vi "Auto Aim.vi"() -> ()   [LabVIEW 2020]
panel:
  out "Bottom Motor":dbl
  out "Top Motor":dbl
  out "Reference":dbl[](array[numeric])
  out "Percent":dbl
  out "Index":i32
  out "Closest":dbl
  in  "Distance":dbl
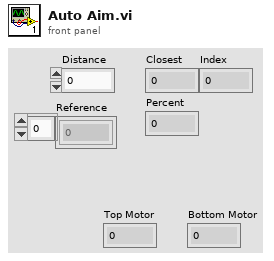
[diagram p1: front panel]
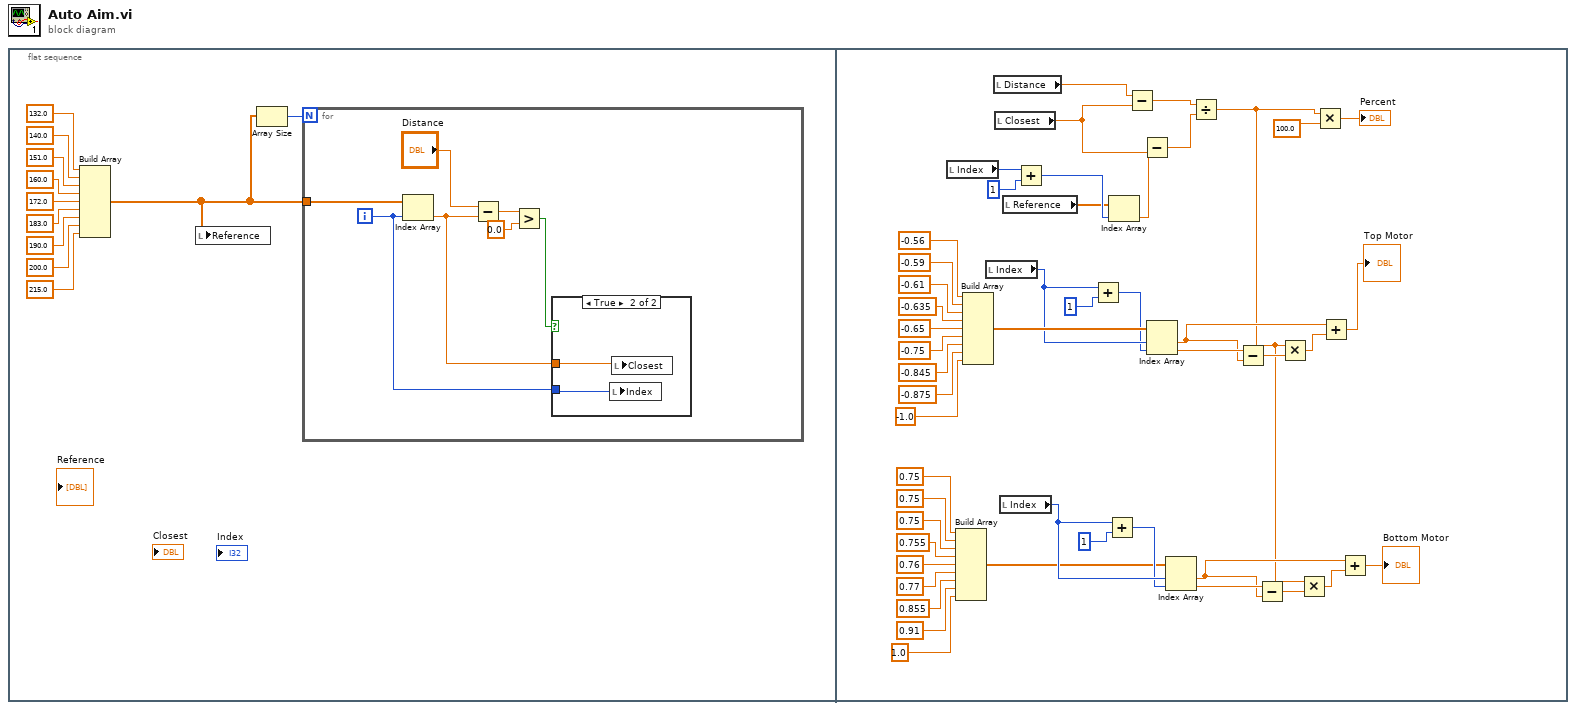
[diagram p0: block diagram]
diagram:
  n1 = flat-sequence {
    frame #0 {
      n2 = Build Array(132.0 ("element"), 140.0 ("element"), 151.0 ("element"), 160.0 ("element"), 172.0 ("element"), 183.0 ("element"), 190.0 ("element"), 200.0 ("element"), 215.0 ("element")) -> (w1:dbl[])
      n3 = local write "Reference"(w1) -> ()
      n4 = Array Size(array=w1) -> (size(s)=w2:i32)
      n5 = for {
        N: w2 -> [_]
        tunnel: w1 -> [w18]
        i -> [w12]
        n6 = Index Array(array=w18, index=w12) -> (element=w13:dbl)
        n7 = Subtract(x="Distance", y=w13) -> (x-y=w17:dbl)
        n8 = Greater?(x=w17, y=0.0) -> (0:w14:bool)
        n9 = case shown="True" w14 {
          tunnel: w13 -> [_ w20]
          tunnel: w12 -> [_ w19]
          frame False {
          }
          frame True {
            n10 = local write "Index"(w19) -> ()
            n11 = local write "Closest"(w20) -> ()
          }
        }
      }
    }
    frame #1 {
      n12 = local read "Index"() -> (w58:i32)
      n13 = Build Array(0.75 ("element"), 0.75 ("element"), 0.75 ("element"), 0.755 ("element"), 0.76 ("element"), 0.77 ("element"), 0.855 ("element"), 0.91 ("element"), 1.0 ("element")) -> (w25:dbl[])
      n14 = Build Array(-0.56 ("element"), -0.59 ("element"), -0.61 ("element"), -0.635 ("element"), -0.65 ("element"), -0.75 ("element"), -0.845 ("element"), -0.875 ("element"), -1.0 ("element")) -> (w50:dbl[])
      n15 = local read "Index"() -> (w48:i32)
      n16 = local read "Distance"() -> (w59:dbl)
      n17 = local read "Closest"() -> (w52:dbl)
      n18 = local read "Index"() -> (w31:i32)
      n19 = local read "Reference"() -> (w51:dbl[])
      n20 = Add(x=w58, y=1) -> (x+y=w56:i32)
      n21 = Add(x=w48, y=1) -> (x+y=w47:i32)
      n22 = Add(x=w31, y=1) -> (x+y=w30:i32)
      n23 = Index Array(array=w51, index=w56) -> (element=w53:dbl)
      n24 = Subtract(x=w59, y=w52) -> (x-y=w54:dbl)
      n25 = Subtract(x=w53, y=w52) -> (x-y=w55:dbl)
      n26 = Index Array(array=w50, index #1=w48, index #2=w47) -> (element #1=w45:dbl, element #2=w46:dbl)
      n27 = Index Array(array=w25, index #1=w31, index #2=w30) -> (element #1=w28:dbl, element #2=w29:dbl)
      n28 = Divide(x=w54, y=w55) -> (x/y=w22:dbl)
      n29 = Subtract(x=w46, y=w45) -> (x-y=w44:dbl)
      n30 = Subtract(x=w29, y=w28) -> (x-y=w27:dbl)
      n31 = Multiply(x=w22, y=w44) -> (x*y=w43:dbl)
      n32 = Multiply(x=w22, y=w27) -> (x*y=w26:dbl)
      n33 = Multiply(x=w22, y=100.0) -> (x*y=→"Percent":dbl)
      n34 = Add(x=w45, y=w43) -> (x+y=→"Top Motor":dbl)
      n35 = Add(x=w28, y=w26) -> (x+y=→"Bottom Motor":dbl)
    }
  }
